vi "Remove Instance.vi"(8 "error in (no error)":errorcluster, 9 "Object Instance":refnum<data-value>, 10 "Base Class (LabVIEW Object)":refnum<class>, 11 "Lookup Service in":refnum<data-value>) -> (0 "error out":errorcluster, 1 "removed?":bool, 3 "Lookup Service out":refnum<data-value>)   [LabVIEW 2014, in "LVCOOOP.lvlib" / "Lookup API.lvlib" / "Lookup Service.lvclass"]
uses:
  Lookup Service.lvclass
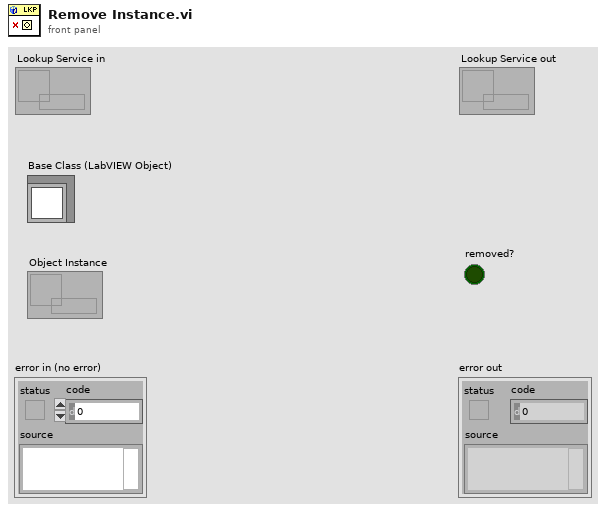
[diagram p1: front panel]
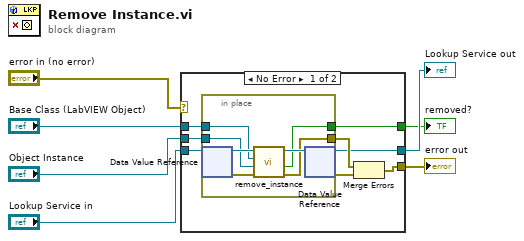
[diagram p0: block diagram]
diagram:
  n1 = case shown="No Error" "error in (no error)" {
    selector: "error in (no error)" -> [_ w24]
    tunnel: [w13 w23] -> w3
    tunnel: [w12 w24] -> w6
    tunnel: "Base Class (LabVIEW Object)" -> [w11 _]
    tunnel: "Object Instance" -> [w10 _]
    tunnel: "Lookup Service in" -> [w9 w23]
    tunnel: [w8 _] -> w1
    frame No Error {
      n2 = in-place {
        in-place-border: [w19] -> w15
        in-place-border: w11 -> [w18]
        in-place-border: w10 -> [w17]
        in-place-border: [w16] -> w8
        n3 = in-place-dvr #1(w9) -> (w22:refnum<class "Lookup Service.lvclass">, w20:errorcluster)
        n4 = call-dynamic "remove_instance.vi"("error in (no error)"=w20, "Object Instance"=w17, "Base Class (LabVIEW Object)"=w18, "Lookup Service in"=w22) -> ("error out"=w19:errorcluster, "removed?"=w16:bool, "Lookup Service out"=w21:refnum<class "Lookup Service.lvclass">)  [unwired: 5 in]
        n5 = in-place-dvr #1(w21) -> (w13:refnum<data-value>, w14:errorcluster)
      }
      n6 = Merge Errors(w15, w14) -> (w12:errorcluster)
    }
    frame Error {
    }
  }
  "error out" <- w6
  "Lookup Service out" <- w3
  "removed?" <- w1
